vi "Limit Testing.vi"   [LabVIEW 2020, in "NI_MAPro.lvlib"]
doc: "Performs limit testing on waveform or cluster input data. The VI compares <B>signal in</B> with <B>upper limit</B> and <B>lower limit</B> and ignores any limit input that is not wired. You can wire <B>output values</B> to a graph to view the limits, signal, and failures. Wire data to the <B>signal in</B> input to determine the polymorphic instance to use or manually select the instance."
uses:
  NI_MAPro.lvlib
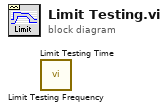
[diagram p0: block diagram]
diagram:
  n1 = call "Limit Testing Frequency.vi"() -> ()  [unwired: 6 in, 6 out]
  n2 = call "Limit Testing Time.vi"() -> ()  [unwired: 6 in, 6 out]
